vi "GEA_Brute_Force.vi"() -> ()   [LabVIEW 2009]
uses:
  <vilib>/Instr/_visa.llb/VISA Configure Serial Port (Instr).vi
panel:
  out "x = y?":bool
  out "unsigned byte array 2":u8[](array[numeric]) format="%.0x"
  in  "Get Hyper Terminal Data":u8[](array[numeric]) format="%.0x"
  out "unsigned byte array":u8[](array[numeric]) format="%.0x"
  in  "VISA resource name":refnum<visa-resource-name>
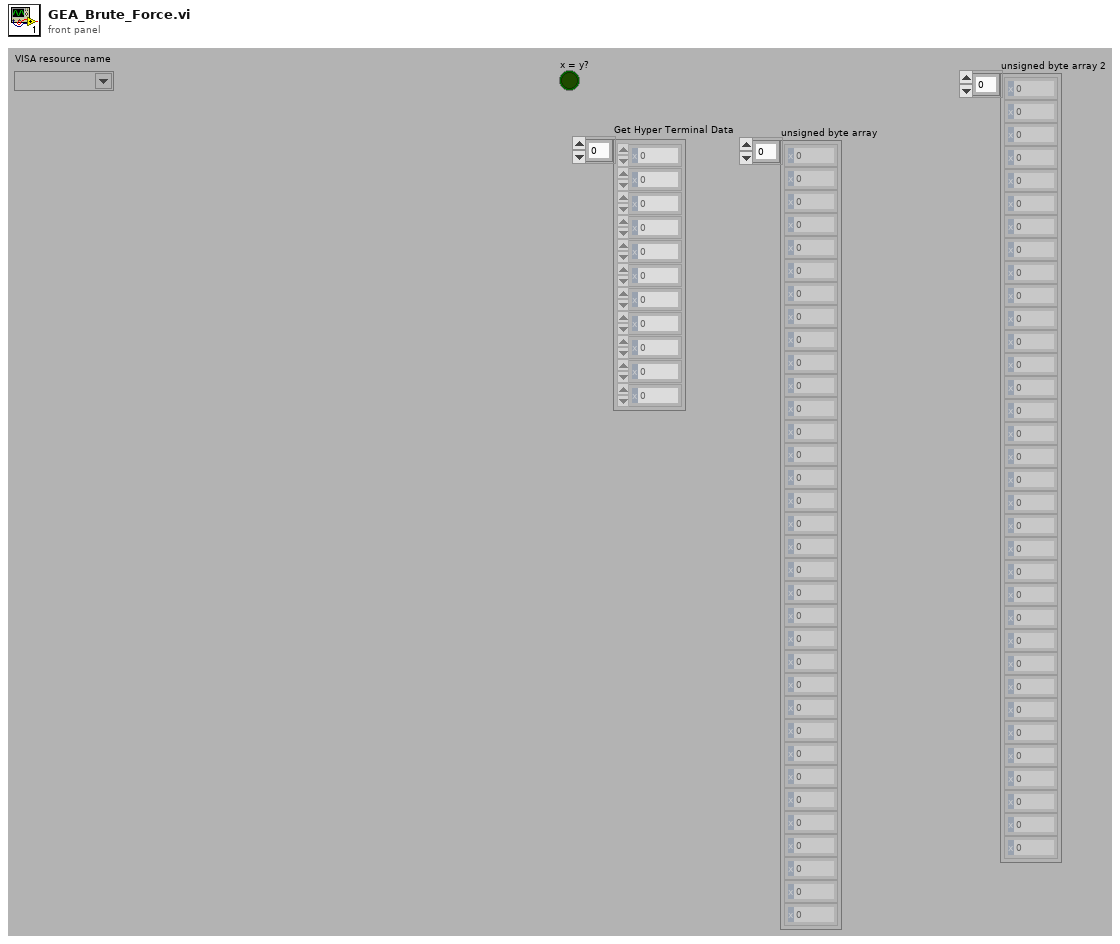
[diagram p1: front panel]
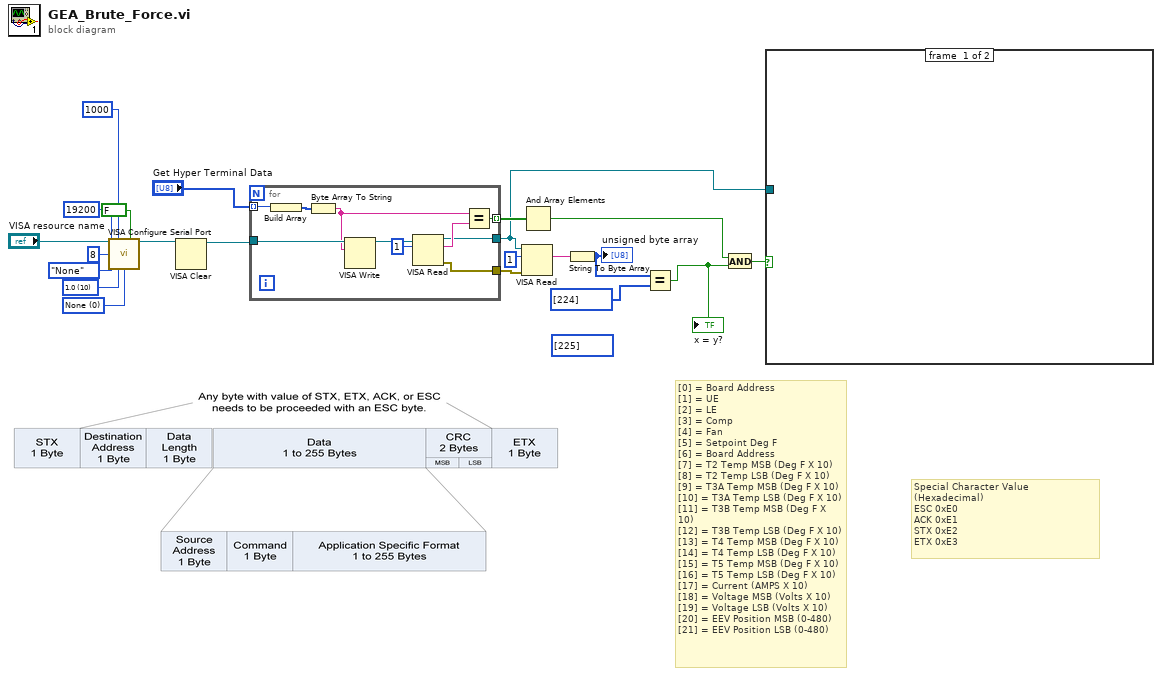
[diagram p0: block diagram]
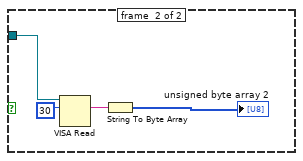
[diagram p2: hidden frame]
diagram:
  w2 = u16 0 items=["None", "XON/XOFF", "RTS/CTS", "XON/XOFF & RTS/CTS", "DTR/DSR", "XON/XOFF & DTR/DSR"] ("flow control (0:none)")
  w3 = u16 10 items=["1.0"=10, "1.5"=15, "2.0"=20] ("stop bits (10: 1 bit)")
  (unwired) u32[] [225]
  # "Special Character\tValue (Hexadecimal)\nESC\t0xE0\nACK\t0xE1\nSTX\t0xE2\nETX\t0xE3"
  # "[0] = Board Address\n[1] = UE\n[2] = LE\n[3] = Comp\n[4] = Fan\n[5] = Setpoint Deg F\n[6] = Board Address\n[7] = T2 Temp MSB (Deg F X 10)\n[8] = T2 Temp LSB (Deg F X 10)\n[9] = T3A Temp MSB (Deg F X 10)\n[10] = T3A Temp LSB (Deg F X 10)\n[11] = T3B Temp MSB (Deg F X 10)\n[12] = T3B Temp LSB (Deg F X 10)\n[13] = T4 Temp MSB (Deg F X 10)\n[14] = T4 Temp LSB (Deg F X 10)\n[15] = T5 Temp MSB (Deg F X 10)\n[16] = T5 Temp LSB (Deg F X 10)\n[17] = Current (AMPS X 10)\n[18] = Voltage MSB (Volts X 10)\n[19] = Voltage LSB (Volts X 10)\n[20] = EEV Position MSB (0-480)\n[21] = EEV Position LSB (0-480)"
  n1 = call-poly "VISA Configure Serial Port"("VISA resource name"="VISA resource name", "timeout (10sec)"=u32 1000, "Enable Termination\nChar (T)"=FALSE ("Enable Termination\nChar (T)"), "baud rate (9600)"=u32 19200, "data bits (8)"=u16 8, "parity (0:none)"=enum16{"None", "Odd", "Even", "Mark", "Space"}."None", "stop bits (10: 1 bit)"=w3, "flow control (0:none)"=w2) -> ("VISA resource name out"=w19:refnum<visa-resource-name>)  [unwired: 6 in, 1 out]
  n2 = VISA Clear(VISA resource name=w19) -> (VISA resource name out=w18:refnum<visa-resource-name>)  [unwired: 1 in, 1 out]
  n3 = for {
    tunnel: w18 -> [w31]
    tunnel: "Get Hyper Terminal Data" -> [w27] mode=indexing
    tunnel: [w24] -> w12 mode=indexing
    tunnel: [w23] -> w17
    tunnel: [w22] -> w7
    n4 = Build Array(w27) -> (w28:u8[])
    n5 = Byte Array To String(unsigned byte array=w28) -> (string=w25:string)
    n6 = VISA Write(VISA resource name=w31, write buffer=w25) -> (VISA resource name out=w30:refnum<visa-resource-name>)  [unwired: 1 in, 2 out]
    n7 = VISA Read(VISA resource name=w30, byte count=u32 1) -> (VISA resource name out=w22:refnum<visa-resource-name>, read buffer=w26:string, error out=w23:errorcluster)  [unwired: 1 in, 1 out]
    n8 = Equal?(x=w25, y=w26) -> (x = y?=w24:bool)
  }
  n9 = VISA Read(VISA resource name=w7, byte count=u32 1, error in (no error)=w17) -> (read buffer=w15:string)  [unwired: 3 out]
  n10 = And Array Elements(Boolean array=w12) -> (logical AND=w11:bool)
  n11 = String To Byte Array(string=w15) -> (unsigned byte array=w10:u8[])
  "unsigned byte array" <- w10
  n12 = Equal?(x=w10, y=u32[] [224]) -> (x = y?=w8:bool)
  "x = y?" <- w8
  n13 = And(x=w11, y=w8) -> (x .and. y?=w13:bool)
  n14 = case shown="True" w13 {
    tunnel: w7 -> [_ w32]
    frame #0 {
    }
    frame #1 {
      n15 = VISA Read(VISA resource name=w32, byte count=u32 30) -> (read buffer=w34:string)  [unwired: 1 in, 3 out]
      n16 = String To Byte Array(string=w34) -> (unsigned byte array=→"unsigned byte array 2":u8[])
    }
  }
